vi "MM9.UpdateUsedObjs.vi"(0 "i ref in":refnum<vi>, 3 "ms timeout (10000)":i32=10000, 5 "error in (no error)":errorcluster) -> (14 "i ref out":refnum<vi>, 16 "UnusedObjs":string[](array[string]), 17 "timed out":bool, 19 "error out":errorcluster)   [LabVIEW 2014, in "MM9.lvlib"]
doc: "This method returns a list of all unused (!) objects updates that list of the used (!) objects in the attribute data."
uses:
  MM9.lvlib
  LEBITLib/LEBITLib.lvlib
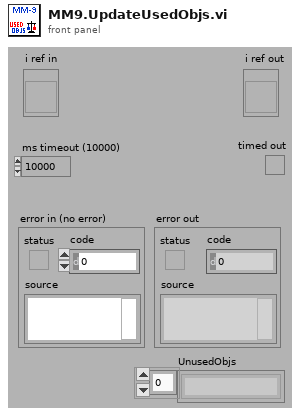
[diagram p1: front panel]
types:
  T1 = typedef "MM9.lvlib/MM9.i attribute.ctl" = cluster{"UsedObjs":string[], "ActScanStep":i32[], "AbortRequest":bool, "StopRequest":bool, "# cycles":i32, "Connected":bool, "MMStatus":T2, "# data":i32, "DIMServices":cluster{"MM6StatusString":string, "MM6StatusID":i32, "discArchiver":string, "discArchiverID":i32, "eventBuilder":string, "eventBuilderID":i32, "GUIIDString":string, "GUIIDStringID":i32}, "dataFile":string, "PGRunning":T3, "ConfigData":T4, "ExtraDataSets":T19}
  T2 = typedef "MM9.lvlib/MM9.status.ctl" = enum16{"loaded", "load_error", "config", "config_error", "init", "init_error", "data_reset", "data_reset_error", "running", "start_error", "run_error", "abort_requested", "aborted", "stop_requested", "stopped", "stop_error", "Connected", "NOTConnected"}
  T3 = typedef "PPG_ABC.lvlib/PPG_ABC.PG_Running.ctl" = i32
  T4 = typedef "LEBITDefs9.lvlib/LEBITDefs.ConfigData.ctl" = cluster{"GenConfig":T5, "Configs":T7[]}
  T5 = typedef "LEBITDefs9.lvlib/LEBITDefs.GenConfig.ctl" = cluster{"Mode":i32, "Logs":T6[]}
  T6 = typedef "LEBITDefs9.lvlib/LEBITDefs.Log.ctl" = cluster{"Name":string, "FctName":string, "Special":string}
  T7 = typedef "LEBITDefs9.lvlib/LEBITDefs.OneConfig.ctl" = cluster{"MCA":T8, "Timing":T9, "Scans":T12[], "FreqDevs":T13[], "CleanDev":T14, "NrCycles":i32, "Specials":T16[], "Delays":T17[], "DAC":T18}
  T8 = typedef "LEBITDefs9.lvlib/LEBITDefs.MCA.ctl" = cluster{"Name":string, "Address":string, "NrChannels":i32, "Gate":i32, "NrPipse":i32, "AcqDelay":i32}
  T9 = typedef "LEBITDefs9.lvlib/LEBITDefs.Timing.ctl" = cluster{"TimeTables":cluster{"TimeTable":T10}[], "Memories":T11[], "ScanX":string, "ScanY":string}
  T10 = typedef "LEBITDefs9.lvlib/LEBITDefs.Timetable.ctl" = dbl[]
  T11 = typedef "LEBITDefs9.lvlib/LEBITDefs.Memory.ctl" = cluster{"Device":string, "ExtTrig":bool, "TT2Use":i32, "PatternTable":string[]}
  T12 = typedef "LEBITDefs9.lvlib/LEBITDefs.ScanDev.ctl" = cluster{"Name":string, "FctName":string, "Values":dbl[], "NrScanVals":i32, "Special":string}
  T13 = typedef "LEBITDefs9.lvlib/LEBITDefs.FreqDev.ctl" = cluster{"Name":string, "Amp":dbl, "CenterFreq":dbl, "Time":dbl}
  T14 = typedef "LEBITDefs9.lvlib/LEBITDefs.CleanDev.ctl" = cluster{"Name":string, "CleanData":T15[]}
  T15 = typedef "LEBITDefs9.lvlib/LEBITDefs.CleanDataType.ctl" = cluster{"Amp":dbl, "Center":dbl, "Plus":dbl, "Minus":dbl, "Time":dbl}
  T16 = typedef "LEBITDefs9.lvlib/LEBITDefs.Special.ctl" = cluster{"Name":string, "FctName":string, "VerySpecial":string, "Data":dbl}
  T17 = typedef "LEBITDefs9.lvlib/LEBITDefs.Delay.ctl" = cluster{"Name":string, "Delay":dbl}
  T18 = typedef "LEBITDefs9.lvlib/LEBITDefs.DAC.ctl" = cluster{"Name":string, "Step1":i32, "Step2":i32}
  T19 = typedef "LEBITDefs9.lvlib/LEBITDefs.ExtraData.ctl" = cluster{"Ions":cluster{"ExcitIonMass":string, "ExcitIonCharge":i32, "CleanIons":cluster{"CleanIonMass":string, "CleanIonCharge":i32}[]}, "TimingDescription":cluster{"TimeTableDescription":cluster{"Times":string[]}[], "PatternTableDescription":cluster{"Pattern":string[]}[]}, "ScanUnits":string[]}[]
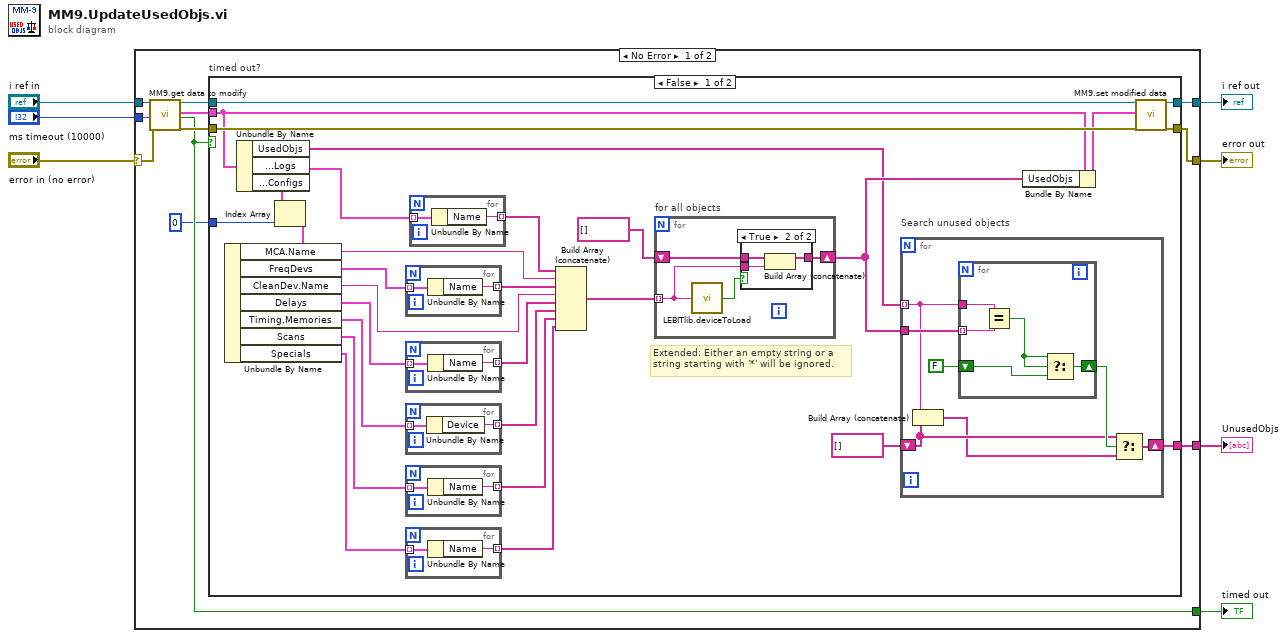
[diagram p0: block diagram]
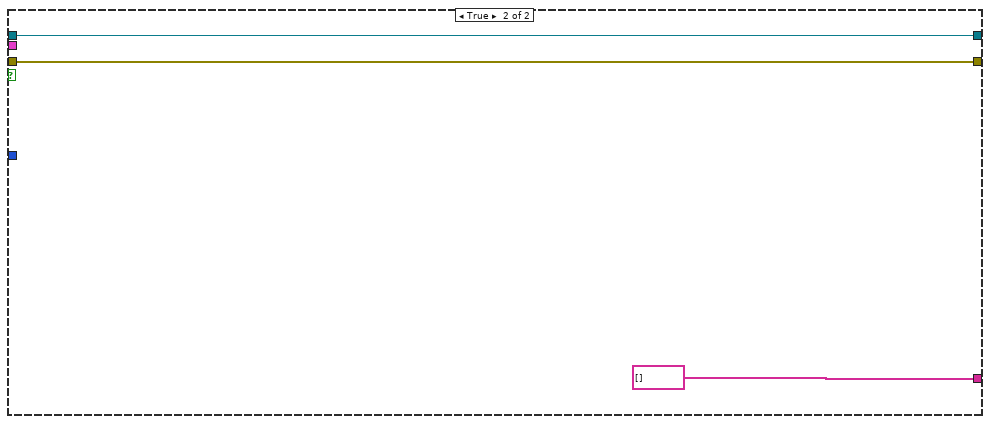
[diagram p3: hidden frame]
diagram:
  n1 = case shown="No Error" "error in (no error)" {
    selector: "error in (no error)" -> [w8 w83]
    tunnel: "i ref in" -> [w18 w84]
    tunnel: [w17 w83] -> w6
    tunnel: [w16 w84] -> w5
    tunnel: "ms timeout (10000)" -> [w12 _]
    tunnel: [w11 _] -> w3
    tunnel: [w10 _] -> w2
    frame No Error {
      n2 = call "MM9.get data to modify.vi"("i ref in"=w18, "ms timeout (10000)"=w12, "error in (no error)"=w8) -> ("i ref out"=w15:refnum<vi>, "i attribute"=w13:T1, "timed out"=w11:bool, "error out"=w14:errorcluster)  [unwired: 13 in]
      n3 = case "timed out?" shown="False" w11 {
        tunnel: [w47 w81] -> w17
        tunnel: [w46 w82] -> w16
        tunnel: w15 -> [w45 w82]
        tunnel: w14 -> [w44 w81]
        tunnel: w13 -> [w42 _]
        tunnel: [w33 string[] []] -> w10
        tunnel: 0 ("index") -> [w23 _]
        frame False {
          # "Extended: Either an empty string or a\nstring starting with '*' will be ignored."
          n4 = Unbundle By Name(w42) -> ("UsedObjs"=w21:string[], "ConfigData.GenConfig.Logs"=w20:T6[], "ConfigData.Configs"=w24:T7[])
          n5 = Index Array(array=w24, index=w23) -> (element=w22:T7)
          n6 = Unbundle By Name(w22) -> ("MCA.Name"=w41:string, "FreqDevs"=w32:T13[], "CleanDev.Name"=w29:string, "Delays"=w39:T17[], "Timing.Memories"=w38:T11[], "Scans"=w37:T12[], "Specials"=w36:T16[])
          n7 = for {
            tunnel: w32 -> [w51] mode=indexing
            tunnel: [w50] -> w31 mode=indexing
            n8 = Unbundle By Name(w51) -> ("Name"=w50:string)
          }
          n9 = for {
            tunnel: w39 -> [w71] mode=indexing
            tunnel: [w70] -> w28 mode=indexing
            n10 = Unbundle By Name(w71) -> ("Name"=w70:string)
          }
          n11 = for {
            tunnel: w38 -> [w69] mode=indexing
            tunnel: [w68] -> w27 mode=indexing
            n12 = Unbundle By Name(w69) -> ("Device"=w68:string)
          }
          n13 = for {
            tunnel: w37 -> [w67] mode=indexing
            tunnel: [w66] -> w26 mode=indexing
            n14 = Unbundle By Name(w67) -> ("Name"=w66:string)
          }
          n15 = for {
            tunnel: w36 -> [w65] mode=indexing
            tunnel: [w64] -> w30 mode=indexing
            n16 = Unbundle By Name(w65) -> ("Name"=w64:string)
          }
          n17 = for {
            tunnel: w20 -> [w49] mode=indexing
            tunnel: [w48] -> w19 mode=indexing
            n18 = Unbundle By Name(w49) -> ("Name"=w48:string)
          }
          n19 = Build Array (concatenate)(w19, w41, w31, w29, w28, w27, w26, w30) -> (w40:string[])
          n20 = for "for all objects" {
            tunnel: w40 -> [w73] mode=indexing
            shift-right: [w74] -> w35
            shift-left: string[] [] -> [w75]
            n21 = call "LEBITlib.deviceToLoad.vi"("DeviceName"=w73) -> ("DeviceIsToLoad"=w72:bool)
            n22 = case shown="True" w72 {
              tunnel: w73 -> [_ w79]
              tunnel: w75 -> [w76 w78]
              tunnel: [w76 w77] -> w74
              frame False {
              }
              frame True {
                n23 = Build Array (concatenate)(w78, w79) -> (w77:string[])
              }
            }
          }
          n24 = for "Search unused objects" {
            tunnel: w21 -> [w54] mode=indexing
            tunnel: w35 -> [w58]
            shift-right: [w55] -> w33
            shift-left: string[] [] -> [w53]
            n25 = Build Array (concatenate)(w54, w53) -> (w52:string[])
            n26 = for {
              tunnel: w54 -> [w63]
              tunnel: w58 -> [w62] mode=indexing
              shift-right: [w59] -> w56
              shift-left: FALSE -> [w60]
              n27 = Equal?(x=w63, y=w62) -> (x = y?=w61:bool)
              n28 = Select(t=w61, s=w61, f=w60) -> (s? t:f=w59:bool)
            }
            n29 = Select(t=w53, s=w56, f=w52) -> (s? t:f=w55:string[])
          }
          n30 = Bundle By Name(cluster=w42, "UsedObjs"=w35) -> (w43:T1)
          n31 = call "MM9.set modified data.vi"("i ref in"=w45, "i attribute"=w43, "error in (no error)"=w44) -> ("i ref out"=w46:refnum<vi>, "error out"=w47:errorcluster)  [unwired: 15 in]
        }
        frame True {
        }
      }
    }
    frame Error {
    }
  }
  "error out" <- w6
  "i ref out" <- w5
  "timed out" <- w3
  "UnusedObjs" <- w2
